vi "CAN Reset.vi"(11 "Channel in":u16) -> (2 "Channel out":u16, 3 "function return":u32)   [LabVIEW 2020, in "PCANBasic.lvlib"]
doc: "TPCANStatus __stdcall CAN_Reset(\n TPCANHandle Channel);"
uses:
  PCANBasic.lvlib
  <userlib>/PCANBasic/PCANBasic.dll
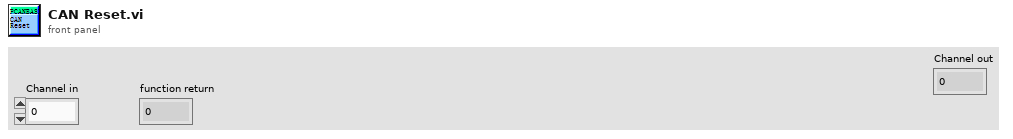
[diagram p1: front panel]
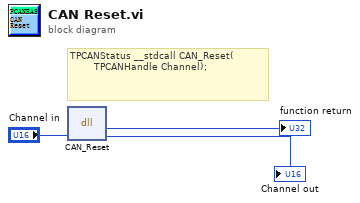
[diagram p0: block diagram]
diagram:
  # "TPCANStatus __stdcall CAN_Reset(\n        TPCANHandle Channel);"
  n1 = dll-call lib="D:/Program Files (x86)/National Instruments/LabVIEW 2020/user.lib/PCANBasic/PCANBasic.dll" fn="CAN_Reset"("Channel"="Channel in") -> ("返回类型"=→"function return":u32, "Channel"=→"Channel out":u16)  [unwired: 3 in, 2 out]
